vi "Metronome.vi"() -> ()   [LabVIEW 2014]
panel:
  in  "ztop":bool
  in  "Beatz Per Minute":dbl
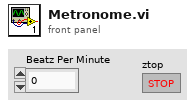
[diagram p1: front panel]
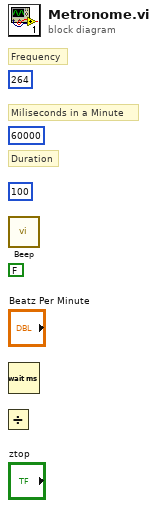
[diagram p0: block diagram]
diagram:
  (unwired) FALSE ("use system alert? (T)")
  (unwired) u32 100 ("duration (msec)")
  (unwired) u32 264 ("frequency (Hz)")
  (unwired) 60000
  # "Duration"
  # "Frequency"
  # "Miliseconds in a Minute"
  n1 = Divide() -> ()  [unwired: 2 in, 1 out]
  n2 = call <vilib>:"Beep.vi"() -> ()  [unwired: 12 in]
  n3 = Wait (ms)() -> ()  [unwired: 1 in, 1 out]
